vi "Numeric Array to String.vi"(11 "Numeric Array":dbl[](array[numeric])) -> (3 "Output String":string)   [LabVIEW 2018, in "Agilent PSG MXG Series.lvlib"]
doc: "Converts numeric array to string with separator , between each element."
uses:
  Agilent PSG MXG Series.lvlib
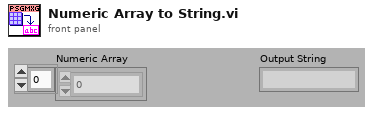
[diagram p1: front panel]
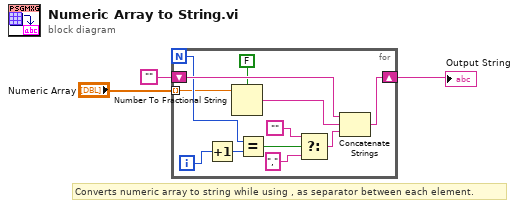
[diagram p0: block diagram]
diagram:
  # "Converts numeric array to string while using , as separator between each element."
  n1 = for {
    N -> [w14]
    tunnel: "Numeric Array" -> [w5] mode=indexing
    shift-right: [w7] -> w2
    shift-left: "" -> [w15]
    i -> [w12]
    n2 = Increment(x=w12) -> (x+1=w13:i32)
    n3 = Number To Fractional String(use system decimal point (T)=FALSE, number=w5) -> (F-format string=w6:string)  [unwired: 2 in]
    n4 = Equal?(x=w14, y=w13) -> (x = y?=w8:bool)
    n5 = Select(t="", s=w8, f="," ("string")) -> (s? t:f=w9:string)
    n6 = Concatenate Strings(w15, w6, w9) -> (w7:string)
  }
  "Output String" <- w2
